vi "Install startup application.vi"(8 "error in (no error)":errorcluster, 10 "Application export directory":path, 11 "RT Management in":refnum<class "RT Management.lvclass">) -> (0 "error out":errorcluster, 3 "RT Management out":refnum<class "RT Management.lvclass">)   [LabVIEW 2016, in "RT Management.lvlib" / "RT Management.lvclass"]
doc: "Installs the RT application located at the \"Application export directory\" to the target, sets the appropriate ni-rt.ini key. This VI does not restart the target.\n\nThe \"Application export directory\" should be the directory containing the \"c\" directory for VxWorks and PharLap and the directory containing the \"home\" directory for Linux RT. Both of these directories should contain the depinstr.bin, which is an easy way to know you are passing in the correct directory path."
uses:
  RT Management.lvclass
  controls/INI key.ctl
  File Transfer Behavior/File Transfer Behavior.lvclass
  RT Management.lvlib
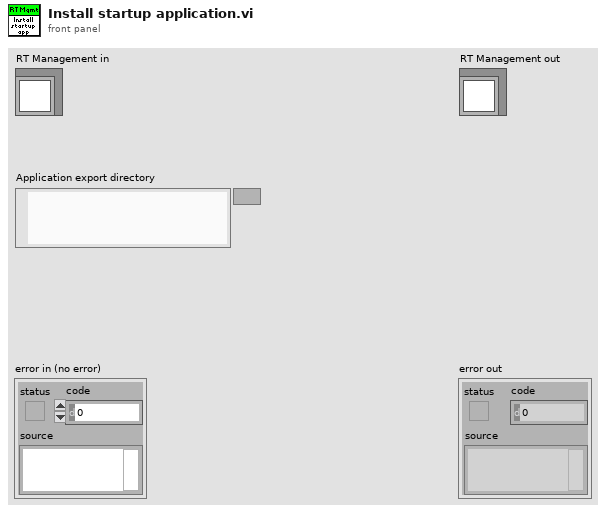
[diagram p1: front panel]
types:
  T1 = typedef "RT Management.lvlib/INI key.ctl" = cluster{"Section":string, "Key name":string, "Key value":string}
  T2 = typedef "RT Management.lvlib/RT Management.lvclass/Operating system.ctl" = enum16{"Unknown", "VxWorks", "PharLap", "Linux-ARM", "Linux-x64"}
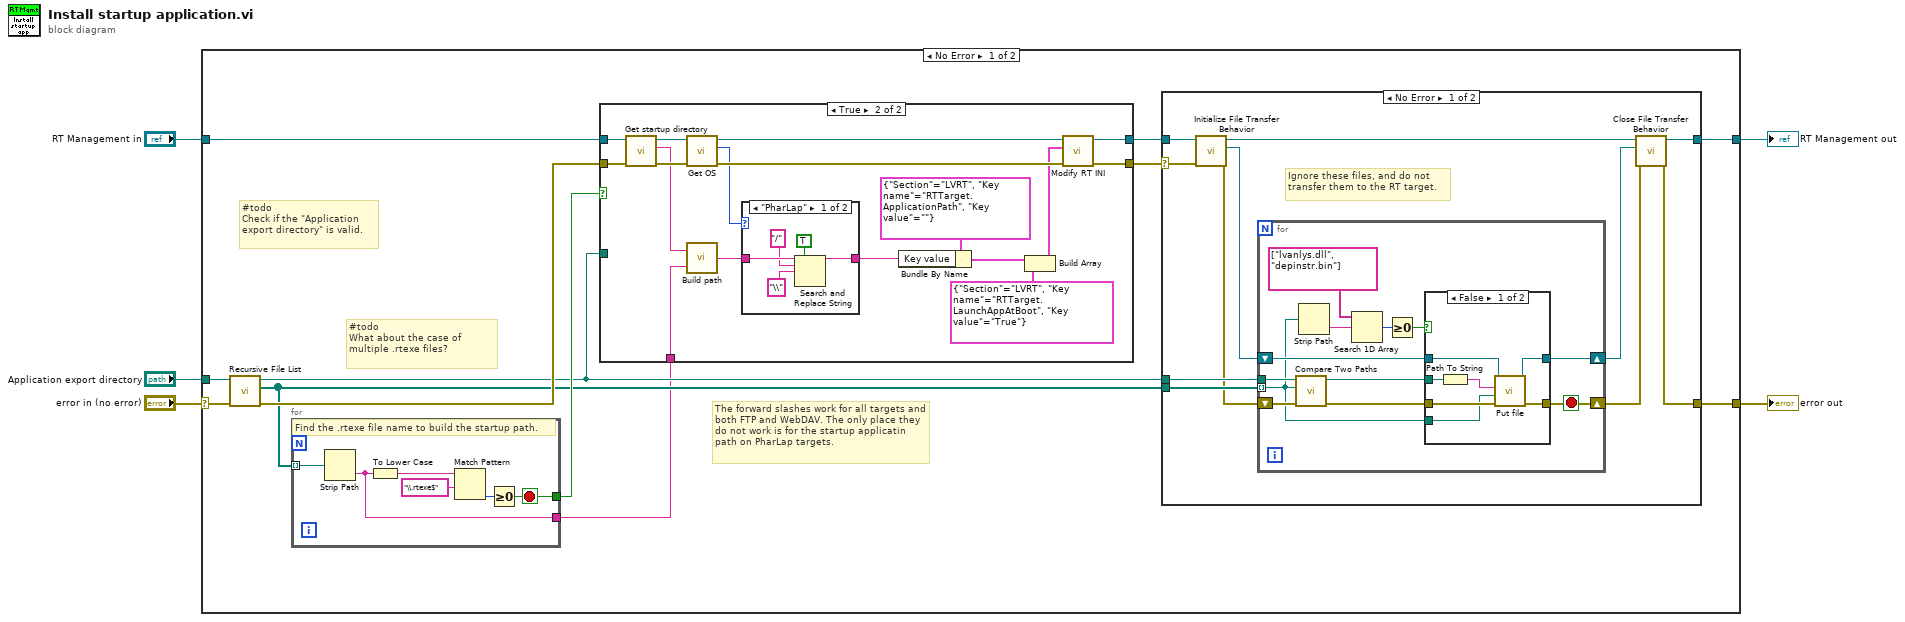
[diagram p0: block diagram]
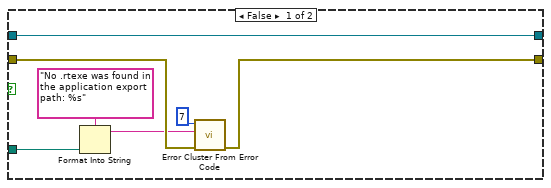
[diagram p4: hidden frame]
diagram:
  n1 = case shown="No Error" "error in (no error)" {
    selector: "error in (no error)" -> [w12 w89]
    tunnel: [w15 w89] -> w4
    tunnel: [w14 w88] -> w2
    tunnel: "RT Management in" -> [w9 w88]
    tunnel: "Application export directory" -> [w17 _]
    frame No Error {
      # "#todo\nCheck if the \"Application export directory\" is valid."
      # "The forward slashes work for all targets and both FTP and WebDAV. The only place they do not work is for the startup applicatin path on PharLap targets."
      # "#todo\nWhat about the case of multiple .rtexe files?"
      n2 = call <vilib>:"Recursive File List.vi"("error in (no error)"=w12, "Folder Path"=w17) -> ("error out"=w10:errorcluster, "All Files in Dir"=w8:path[], "dup Folder Path"=w7:path)  [unwired: 5 in, 2 out]
      n3 = for {
        tunnel: w8 -> [w87] mode=indexing
        tunnel: [w83] -> w6
        tunnel: [w82] -> w13
        stop <- w82 stop-if-true
        # "Find the .rtexe file name to build the startup path."
        n4 = Strip Path(path=w87) -> (name=w83:string)  [unwired: 1 out]
        n5 = To Lower Case(string=w83) -> (all lower case string=w86:string)
        n6 = Match Pattern(string=w86, regular expression="\\.rtexe$") -> (offset past match=w84:i32)  [unwired: 1 in, 3 out]
        n7 = Greater Or Equal To 0?(x=w84) -> (x >= 0?=w82:bool)
      }
      n8 = case shown="True" w13 {
        tunnel: w9 -> [w57 w68]
        tunnel: w10 -> [w58 w67]
        tunnel: [w57 w74] -> w16
        tunnel: [w52 w70] -> w11
        tunnel: w7 -> [w54 _]
        tunnel: w6 -> [_ w62]
        frame False {
          n9 = Format Into String(format string="No .rtexe was found in the application export path: %s" ("error message (\"\")"), w54) -> (resulting string=w53:string)  [unwired: 2 in, 1 out]
          n10 = call <vilib>:"Error Cluster From Error Code.vi"("error in (no error)"=w58, "error message (\"\")"=w53, "error code (0)"=7) -> ("error out"=w52:errorcluster)  [unwired: 6 in]
        }
        frame True {
          n11 = call "Get startup directory.vi"("error in (no error)"=w67, "RT Management in"=w68) -> ("error out"=w66:errorcluster, "Startup directory"=w61:string, "RT Management out"=w65:refnum<class "RT Management.lvclass">)  [unwired: 7 in]
          n12 = call "Get OS.vi"("error in (no error)"=w66, "RT Management in"=w65) -> ("error out"=w75:errorcluster, "Operating System"=w60:T2, "RT Management out"=w64:refnum<class "RT Management.lvclass">)  [unwired: 6 in, 1 out]
          n13 = call "Build path.vi"("Relative path"=w62, "Base path"=w61) -> ("Resulting path"=w63:string)
          n14 = case shown="\"PharLap\"" w60 {
            tunnel: w63 -> [w80 w81]
            tunnel: [w76 w81] -> w59
            frame "PharLap" {
              n15 = Search and Replace String(replace all?=TRUE ("replace all? (F)"), input string=w80, search string="/", replace string="\\" ("replace string (\"\")")) -> (result string=w76:string)  [unwired: 4 in, 3 out]
            }
            frame Default {
            }
          }
          n16 = Bundle By Name(cluster=T1 {"Section"="LVRT", "Key name"="RTTarget.ApplicationPath", "Key value"=""} ("INI_Key"), "Key value"=w59) -> (w72:T1)
          n17 = Build Array(w72, T1 {"Section"="LVRT", "Key name"="RTTarget.LaunchAppAtBoot", "Key value"="True"} ("element")) -> (w71:T1[])
          n18 = call "Modify RT INI.vi"("error in (no error)"=w75, "Keys to edit"=w71, "RT Management in"=w64) -> ("error out"=w70:errorcluster, "RT Management out"=w74:refnum<class "RT Management.lvclass">)  [unwired: 7 in]
        }
      }
      n19 = case shown="No Error" w11 {
        selector: w11 -> [w22 w50]
        tunnel: w16 -> [w23 w51]
        tunnel: [w27 w50] -> w15
        tunnel: [w26 w51] -> w14
        tunnel: w7 -> [w25 _]
        tunnel: w8 -> [w24 _]
        frame No Error {
          # "Ignore these files, and do not transfer them to the RT target."
          n20 = call "Initialize File Transfer Behavior.vi"("error in (no error)"=w22, "RT Management in"=w23) -> ("error out"=w20:errorcluster, "File Transfer Behavior out"=w21:refnum<class "File Transfer Behavior.lvclass">, "RT Management out"=w19:refnum<class "RT Management.lvclass">)  [unwired: 7 in]
          n21 = for {
            tunnel: w24 -> [w35] mode=indexing
            shift-right: [w30] -> w28
            shift-left: w20 -> [w40]
            tunnel: w25 -> [w38]
            shift-right: [w37] -> w18
            shift-left: w21 -> [w36]
            stop <- w30 stop-if-true
            n22 = call <vilib>:"Compare Two Paths.vi"("error in (no error)"=w40, "Path 2"=w35, "Path 1"=w38) -> ("error out"=w29:errorcluster, "Relative Path from 1 to 2"=w39:path)  [unwired: 5 in, 2 out]
            n23 = Strip Path(path=w35) -> (name=w31:string)  [unwired: 1 out]
            n24 = Search 1D Array(1D array=string[] ["lvanlys.dll", "depinstr.bin"], element=w31) -> (index of element=w34:i32)  [unwired: 1 in]
            n25 = Greater Or Equal To 0?(x=w34) -> (x >= 0?=w32:bool)
            n26 = case shown="False" w32 {
              tunnel: w39 -> [w47 _]
              tunnel: [w46 w48] -> w30
              tunnel: [w45 w49] -> w37
              tunnel: w36 -> [w43 w49]
              tunnel: w29 -> [w42 w48]
              tunnel: w35 -> [w41 _]
              frame False {
                n27 = Path To String(path=w47) -> (string=w44:string)
                n28 = call-dynamic "Put file.vi"("error in (no error)"=w42, "Local path"=w41, "Remote path"=w44, "File Transfer Behavior in"=w43) -> ("error out"=w46:errorcluster, "File Transfer Behavior out"=w45:refnum<class "File Transfer Behavior.lvclass">)  [unwired: 6 in]
              }
              frame True {
              }
            }
          }
          n29 = call "Close File Transfer Behavior.vi"("error in (no error)"=w28, "File Transfer Behavior in"=w18, "RT Management in"=w19) -> ("error out"=w27:errorcluster, "RT Management out"=w26:refnum<class "RT Management.lvclass">)  [unwired: 7 in]
        }
        frame Error {
        }
      }
    }
    frame Error {
    }
  }
  "error out" <- w4
  "RT Management out" <- w2
